vi "svx_DAQ_CreateChannelName.vi"(11 "DAQmx Channel In":tag) -> (1 "Channel Name":string, 3 "DAQmx Channel Out":tag)   [LabVIEW 2017, in "SVX NI-DAQmx AI Configuration XControl.xctl"]
uses:
  <vilib>/addons/Sound and Vibration/svt_DAQmx/Configuration XControl/SVX NI-DAQmx AI Configuration XControl.xctl
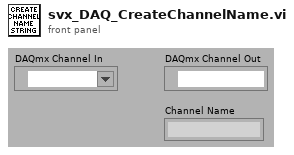
[diagram p1: front panel]
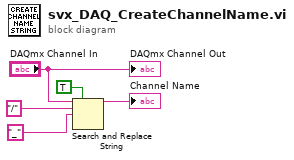
[diagram p0: block diagram]
diagram:
  n1 = Search and Replace String(replace all?=TRUE ("replace all? (F)"), input string="DAQmx Channel In", search string="/", replace string="_" ("replace string (\"\")")) -> (result string=→"Channel Name":string)  [unwired: 4 in, 3 out]
  "DAQmx Channel Out" <- "DAQmx Channel In"
